vi "c_to_f.vi"(11 "*C Thermometer":dbl) -> (3 "Numeric":dbl)   [LabVIEW 2015]
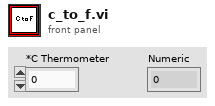
[diagram p1: front panel]
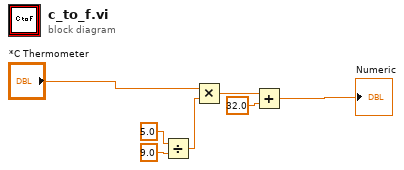
[diagram p0: block diagram]
diagram:
  n1 = Divide(x=5.0, y=9.0) -> (x/y=w4:dbl)
  n2 = Multiply(x="*C Thermometer", y=w4) -> (x*y=w5:dbl)
  n3 = Add(x=w5, y=32.0) -> (x+y=→"Numeric":dbl)
